vi "Write inputs.vi"(5 "inputs":refnum<class "Terminal.lvclass">[](array[class]), 9 "FlatSequence in":refnum<class "FlatSequence.lvclass">) -> (3 "FlatSequence out":refnum<class "FlatSequence.lvclass">)   [LabVIEW 2014, in "FlatSequence.lvclass"]
uses:
  FlatSequence.lvclass
  Terminal/Terminal.lvclass
  FlatSequence.lvclass/FlatSequence.ctl
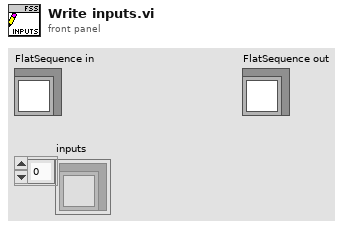
[diagram p1: front panel]
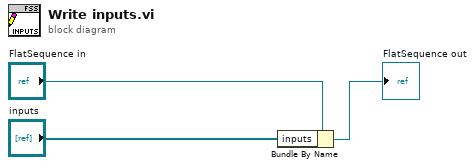
[diagram p0: block diagram]
diagram:
  n1 = Bundle By Name(cluster="FlatSequence in", "inputs"="inputs") -> (→"FlatSequence out":refnum<class "FlatSequence.lvclass">)
